vi "Star Input to Waveform Array.vi"(9 "TagArray":refnum<class "Tag.lvclass">[](array[class]), 10 "InputArray":T1(array[cluster])) -> (2 "Array":dbl[](array[numeric]))   [LabVIEW 2014]
uses:
  Tag.lvclass
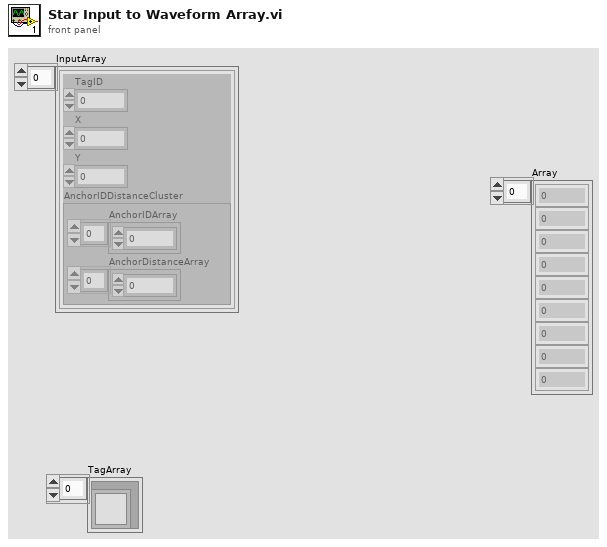
[diagram p1: front panel]
types:
  T1 = cluster{"TagID":dbl, "X":dbl, "Y":dbl, "AnchorIDDistanceCluster":cluster{"AnchorIDArray":dbl[], "AnchorDistanceArray":dbl[]}}[]
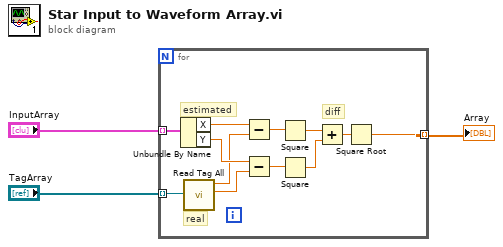
[diagram p0: block diagram]
diagram:
  n1 = for {
    tunnel: "InputArray" -> [w9] mode=indexing
    tunnel: "TagArray" -> [w8] mode=indexing
    tunnel: [w4] -> w2 mode=indexing
    # "diff"
    # "real"
    # "estimated"
    n2 = Unbundle By Name ("estimated xy values")(w9) -> ("X"=w11:dbl, "Y"=w15:dbl)
    n3 = call "Read Tag All.vi"("Tag.lvclass"=w8) -> ("TagY"=w14:dbl, "TagX"=w10:dbl)  [unwired: 5 in, 4 out]
    n4 = Subtract(x=w11, y=w10) -> (x-y=w13:dbl)
    n5 = Subtract(x=w15, y=w14) -> (x-y=w12:dbl)
    n6 = Square(x=w13) -> (x^2=w6:dbl)
    n7 = Square(x=w12) -> (x^2=w5:dbl)
    n8 = Add(x=w6, y=w5) -> (x+y=w7:dbl)
    n9 = Square Root(x=w7) -> (sqrt(x)=w4:dbl)
  }
  "Array" <- w2
